vi "ReadFifo.vi"(8 "error in (no error)":errorcluster, 10 "N":i32, 11 "FPGA_Interface in":refnum<class "FPGA_Interface.lvclass">) -> (0 "error out":errorcluster, 2 "Data":dbl[](array[numeric]), 3 "FPGA_Interface out":refnum<class "FPGA_Interface.lvclass">)   [LabVIEW 2019, in "FPGA_Interface.lvclass"]
uses:
  FPGA_Interface.lvclass
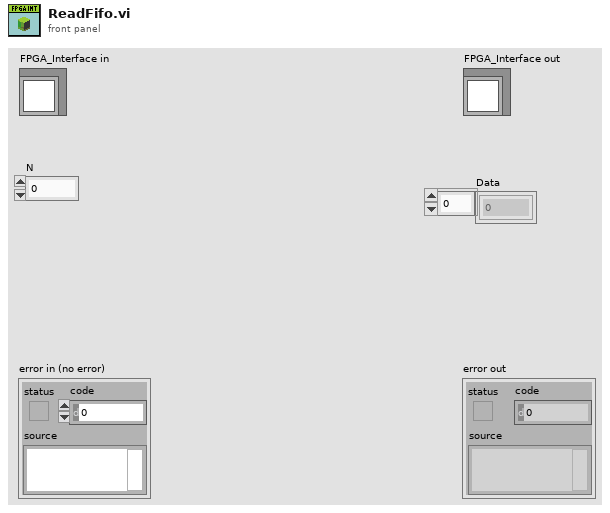
[diagram p1: front panel]
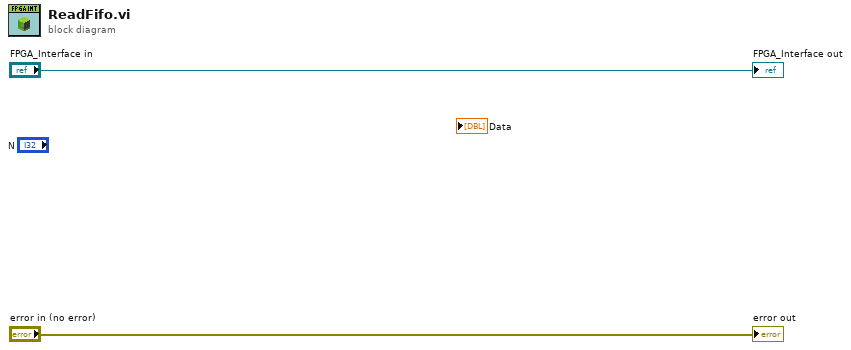
[diagram p0: block diagram]
diagram:
  "error out" <- "error in (no error)"
  "FPGA_Interface out" <- "FPGA_Interface in"
